vi "Write pos_curr.vi"(8 "error in (no error)":errorcluster, 10 "set_pos":dbl[](array[numeric]), 11 "_stage in":refnum<class "_stage.lvclass">) -> (0 "error out":errorcluster, 3 "_stage out":refnum<class "_stage.lvclass">)   [LabVIEW 2019, in "_stage.lvlib" / "_stage.lvclass"]
uses:
  _stage.lvclass
  _stage.lvclass/_stage.ctl
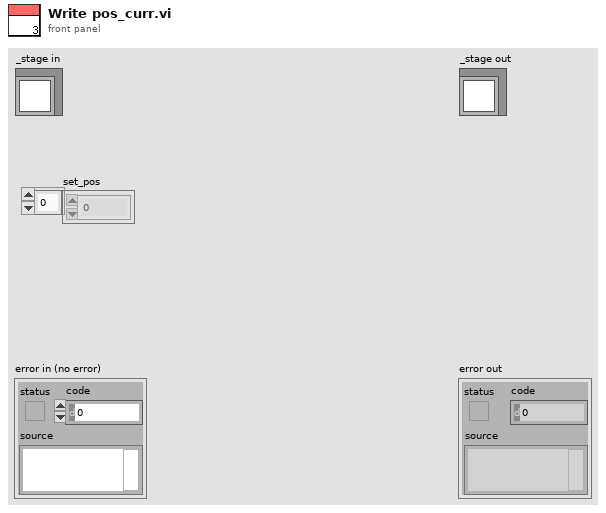
[diagram p1: front panel]
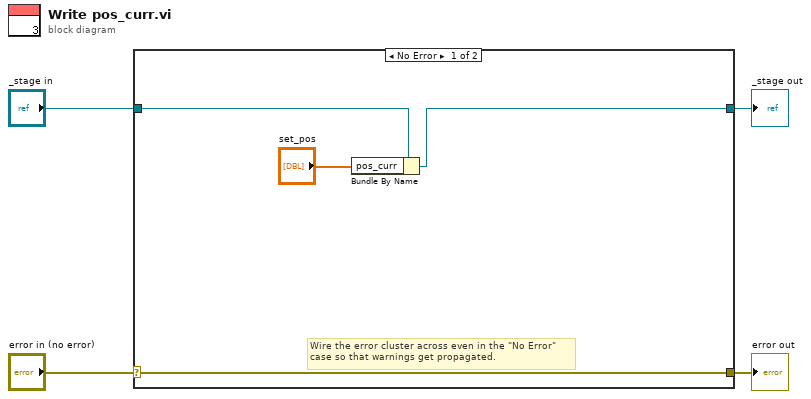
[diagram p0: block diagram]
diagram:
  n1 = case shown="No Error" "error in (no error)" {
    selector: "error in (no error)" -> [w8 w10]
    tunnel: [w8 w10] -> w3
    tunnel: [w6 w9] -> w1
    tunnel: "_stage in" -> [w7 w9]
    frame No Error {
      # "Wire the error cluster across even in the \"No Error\"\ncase so that warnings get propagated."
      n2 = Bundle By Name(cluster=w7, "pos_curr"="set_pos") -> (w6:refnum<class "_stage.lvclass">)
    }
    frame Error {
    }
  }
  "error out" <- w3
  "_stage out" <- w1
